vi "wayne.vi"() -> ()   [LabVIEW 2012]
uses:
  <vilib>/DAQmx/write.llb/DAQmx Write.vi
  <vilib>/DAQmx/write.llb/DAQmx Write (Digital 1D Bool NChan 1Samp 1Line).vi
  <vilib>/DAQmx/miscellaneous.llb/DAQmx Fill In Error Info.vi
  <vilib>/DAQmx/create/channels.llb/DAQmx Create Virtual Channel.vi
  <vilib>/DAQmx/create/channels.llb/DAQmx Create Channel (DO-Digital Output).vi
panel:
  out "inhibit":dbl=10.092000007629395
  out "delay":dbl=11.291999816894531
  in  "delay time (s)":dbl=1.2
  in  "Rolling Average Size":i32=25 min=1 step=1
  in  "inhibit time (s)":dbl=18.0
  in  "ECOLAB Button":bool
  in  "Tab Control":enum32{" GRAPHS   ", "CONFIG"}(tab)
  in  "on pulse simulator":bool
  out "Graph [0]":cluster{"Waveform":dbl, dbl}(graph)={"Waveform"=-0.0019147462699382683, -0.0017572258204325486}
  in  "on threshold (volts)":dbl=0.5
  out "AI":dbl[](array[numeric])=[-0.0017572258204325486] format="%.3f"
  out "DAQ Loop":i32=93368
  in  "DAQ wait ms":u32=3
  out "ON Pulse":bool
  in  "off threshold (volts)":dbl=-0.2
  in  "off pulse simulator":bool
  out "SOAP SIGNAL":bool
  out "Time (s)":dbl
  out "9205 Error":errorcluster
  in  "DAQ Selection":tag="9205/ai0"
  in  "maximum value":dbl=10.0
  in  "minimum value":dbl=-10.0
  out "9481 Error":errorcluster
  in  "9481 Name":tag="9481"
  in  "Relay Control":bool[](array[boolean])=[FALSE, FALSE, FALSE, FALSE]
  in  "Trim HI / LO [%]":dbl=2.0 min=0.0 max=100.0
  in  "Stop Program":bool=TRUE
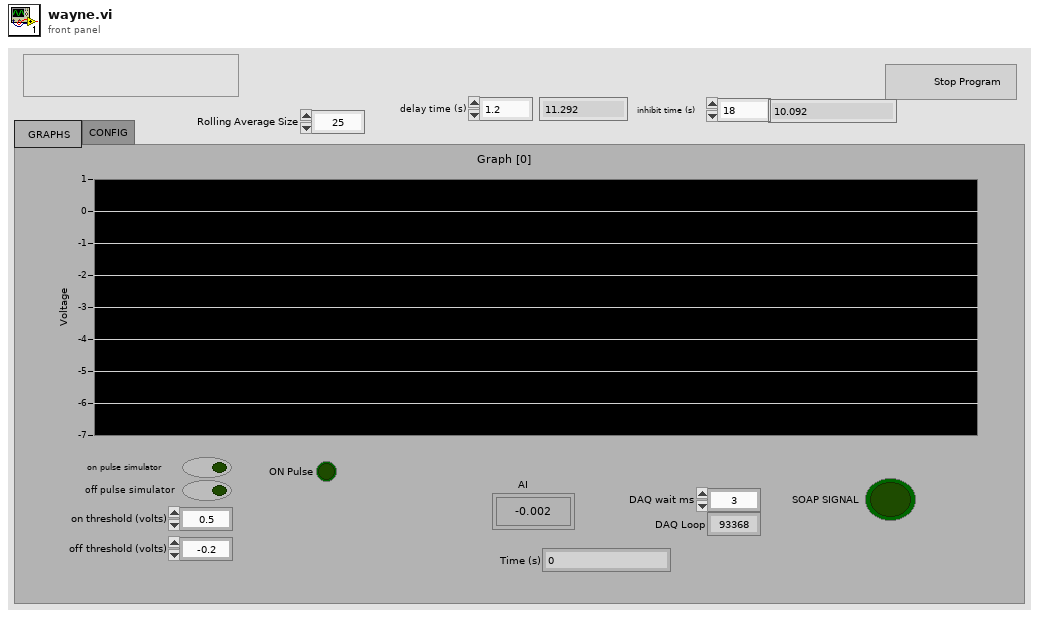
[diagram p1: front panel]
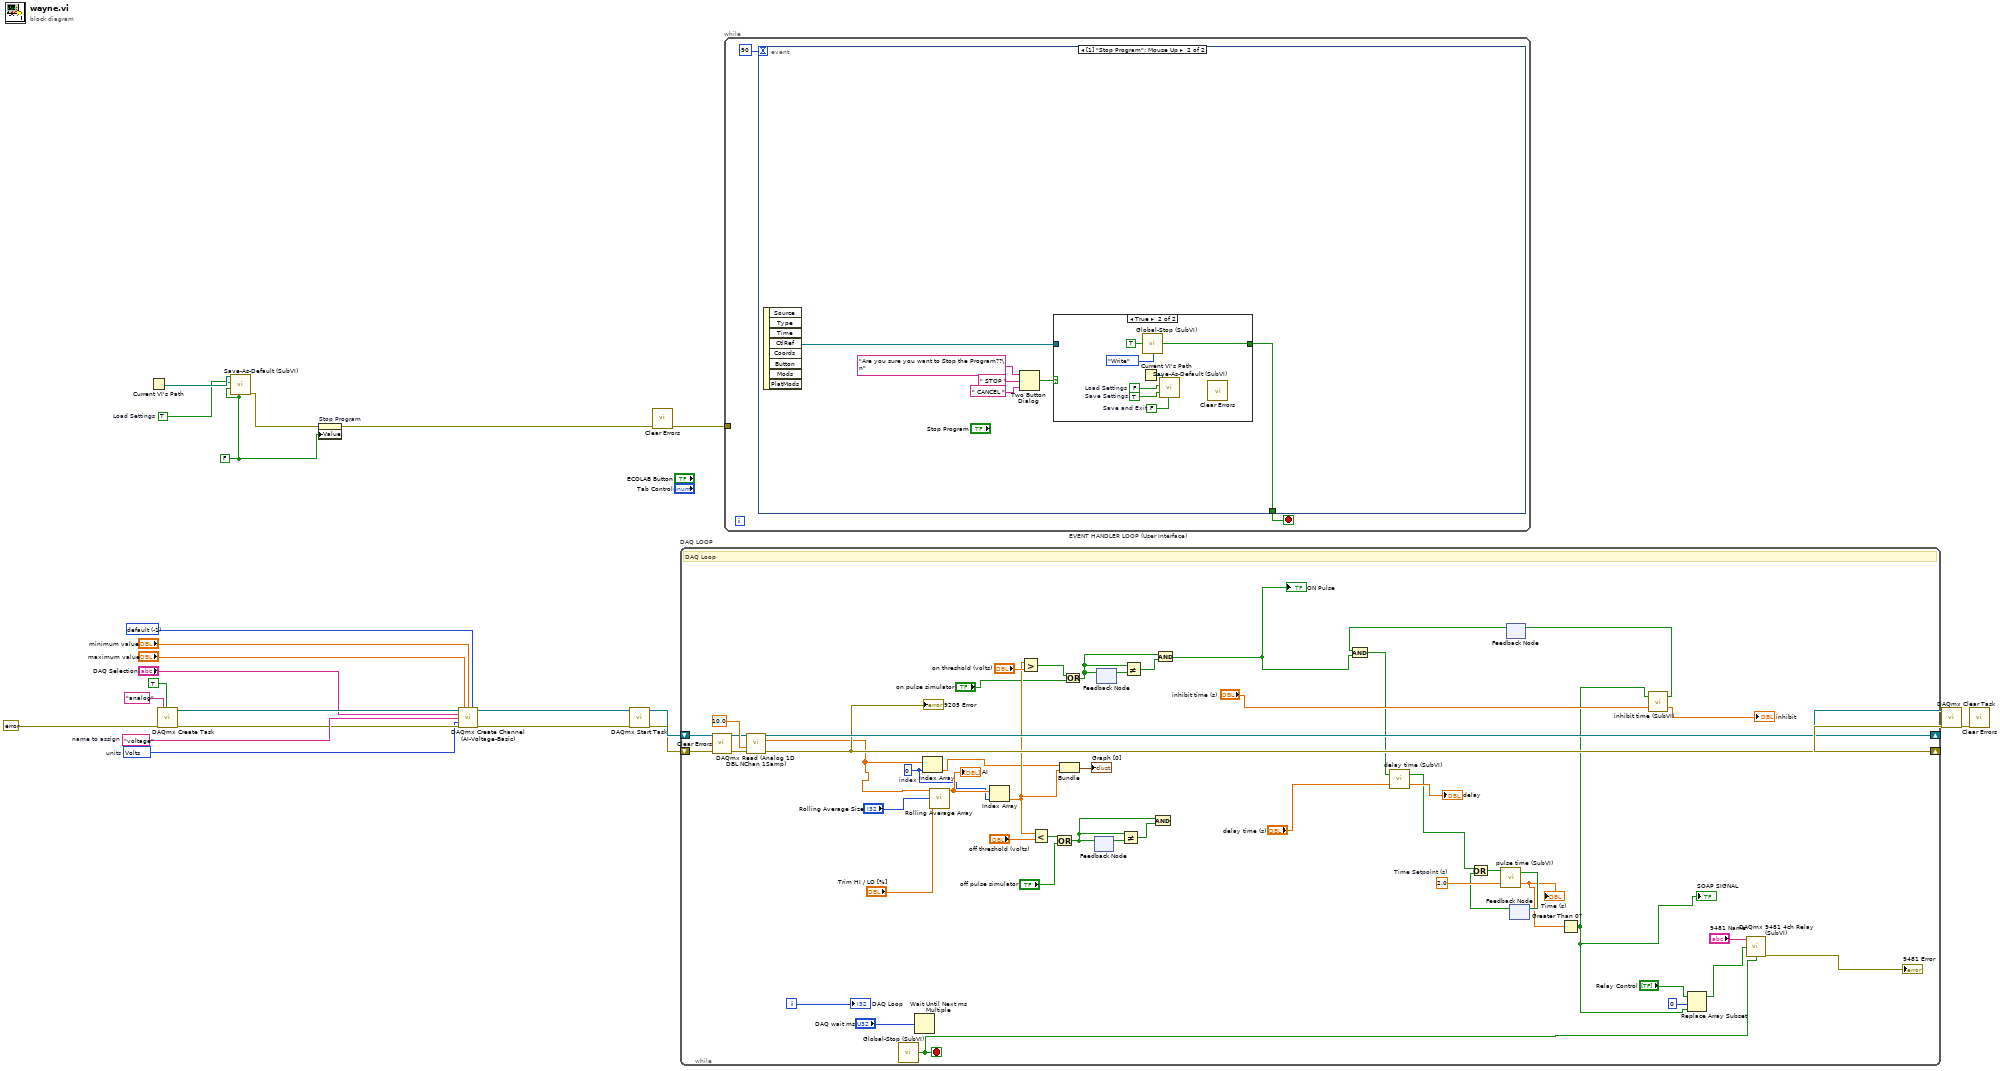
[diagram p0: block diagram]
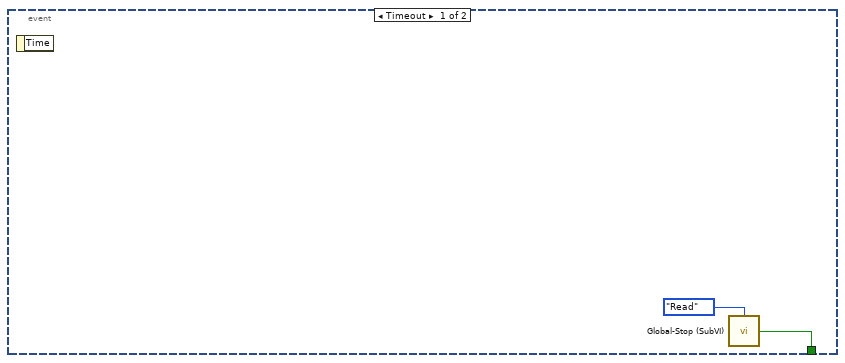
[diagram p2: hidden frame]
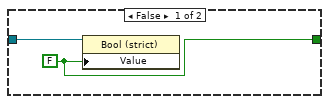
[diagram p3: hidden frame]
diagram:
  w3 = TRUE  # Load Settings
  w6 = 10348 items=["Volts"=10348, "From Custom Scale"=10065]  # units
  w8 = "voltage"  # name to assign
  w1 = FALSE
  w14 = -1 items=["default"=-1, "RSE"=10083, "NRSE"=10078, "Differential"=10106, "Pseudodifferential"=12529]
  n1 = Current VI's Path() -> (path=w4:path)
  n2 = call <vilib>:"DAQmx Create Task.vi"("new task name"="analog", "auto cleanup"=TRUE, "error in"=errorcluster {"status"=FALSE, "code"=0, "source"=""}) -> ("task out"=w13:refnum<k21>, "error out"=w7:errorcluster)  [unwired: 11 in]
  n3 = call "Save-As-Default (SubVI).vi"("Current VI's Path"=w4, "Load Settings"=w3, "Save Settings"=w1, "Save and Exit"=w1) -> ("Save as Default Error"=w2:errorcluster)  [unwired: 15 in]
  n4 = property on="Stop Program" class="Bool (strict)"(error in=w2, "Value"=w1) -> (error out=w17:errorcluster)  [unwired: 1 in, 1 out]
  n5 = call <vilib>:"DAQmx Create Channel (AI-Voltage-Basic).vi"("task in"=w13, "maximum value"="maximum value", "minimum value"="minimum value", "input terminal configuration"=w14, "physical channels"="DAQ Selection", "name to assign"=w8, "units"=w6, "error in"=w7) -> ("task out"=w10:refnum<k21>, "error out"=w9:errorcluster)  [unwired: 6 in]
  n6 = call <vilib>:"DAQmx Start Task.vi"("task/channels in"=w10, "error in"=w9) -> ("task out"=w20:refnum<k21>, "error out"=w18:errorcluster)  [unwired: 12 in]
  n7 = call <vilib>:"Clear Errors.vi"("error in (no error)"=w17) -> ("error out"=w16:errorcluster)  [unwired: 6 out]
  n8 = while "DAQ LOOP" {
    shift-right: [w68] -> w19
    shift-left: w20 -> [w70]
    shift-right: [w67] -> w22
    shift-left: w18 -> [w73]
    i -> [w58]
    stop <- w64 stop-if-true
    w35 = 2.0  # Time Setpoint (s)
    w47 = 0  # index
    # "DAQ Loop"
    n9 = call <vilib>:"Clear Errors.vi"("error in (no error)"=w73) -> ("error out"=w69:errorcluster)  [unwired: 6 in]
    n10 = call <vilib>:"DAQmx Read (Analog 1D DBL NChan 1Samp).vi"("task/channels in"=w70, "timeout"=10.0, "error in"=w69) -> ("task out"=w68:refnum<k21>, "data"=w48:dbl[], "error out"=w67:errorcluster)  [unwired: 10 in]
    "9205 Error" <- w67
    n11 = call "Global-Stop (SubVI).vi"() -> ("OUT"=w64:bool)  [unwired: 4 in]
    n12 = Wait Until Next ms Multiple(millisecond multiple="DAQ wait ms") -> ()  [unwired: 1 out]
    n13 = Index Array(array=w48, index=w47) -> (element=w44:dbl)
    n14 = call "Rolling Average Array.vi"("Raw Signals"=w48, "Rolling Average Size"="Rolling Average Size", "Trim HI / LO [%]"="Trim HI / LO [%]") -> ("Averaged Signals"=w49:dbl[])  [unwired: 12 in]
    "AI" <- w49
    n15 = Index Array(array=w49, index=w47) -> (element=w46:dbl)
    n16 = Greater?(x=w46, y="on threshold (volts)") -> (0:w41:bool)
    n17 = Less?(x=w46, y="off threshold (volts)") -> (x < y?=w54:bool)
    n18 = Or(x=w54, y="off pulse simulator") -> (x .or. y?=w52:bool)
    n19 = Bundle("Waveform"=w44, w46) -> (→"Graph [0]":cluster{"Waveform":dbl, dbl})  [unwired: 1 in]
    n20 = Or(x=w41, y="on pulse simulator") -> (x .or. y?=w40:bool)
    n21 = feedback #1() -> (w59:bool)  [unwired: 1 in]
    n22 = feedback-in #1(w52) -> ()
    n23 = feedback #2() -> (w62:bool)  [unwired: 1 in]
    n24 = feedback-in #2(w40) -> ()
    n25 = Not Equal?(x=w52, y=w59) -> (x != y?=w60:bool)
    n26 = Not Equal?(x=w40, y=w62) -> (x != y?=w43:bool)
    n27 = And(x=w52, y=w60) -> ()  [unwired: 1 out]
    n28 = And(x=w40, y=w43) -> (x .and. y?=w28:bool)
    "ON Pulse" <- w28
    n29 = feedback #3() -> (w26:bool)  [unwired: 1 in]
    n30 = And(x=w26, y=w28) -> (x .and. y?=w27:bool)
    n31 = call "delay time (SubVI).vi"("Time Setpoint (s)"="delay time (s)", "START/RESET TIMER"=w27) -> ("Time (s)"=→"delay":dbl, "Time Elapsed"=w33:bool)
    n32 = feedback #4() -> (w32:bool)  [unwired: 1 in]
    n33 = Or(x=w33, y=w32) -> (x .or. y?=w31:bool)
    n34 = call "pulse time (SubVI).vi"("Time Setpoint (s)"=w35, "START/RESET TIMER"=w31) -> ("Time (s)"=w30:dbl, "Time Elapsed"=w34:bool)
    "Time (s)" <- w30
    n35 = feedback-in #4(w34) -> ()
    n36 = Greater Than 0?(x=w30) -> (x > 0?=w25:bool)
    "SOAP SIGNAL" <- w25
    n37 = call "inhibit time (SubVI).vi"("Time Setpoint (s)"="inhibit time (s)", "START/RESET TIMER"=w25) -> ("Time (s)"=→"inhibit":dbl, "Time Elapsed"=w29:bool)
    n38 = feedback-in #3(w29) -> ()
    n39 = Replace Array Subset(array="Relay Control", new element=w25, index=0) -> (w55:bool[])
    n40 = call "DAQmx 9481 4ch Relay (SubVI).vi"("9481 Name"="9481 Name", "Relay Control"=w55, "Stop Program"=w64) -> ("9481 Error"=→"9481 Error":errorcluster)  [unwired: 12 in]
    "DAQ Loop" <- w58
  }
  n41 = while "EVENT HANDLER LOOP (User Interface)" {
    tunnel: w16 -> [_]
    stop <- w75 stop-if-true
    n42 = event shown="[1] \"Stop Program\": Mouse Up" {
      selector: _ -> [_ _]
      dyn-events: _ -> [_ _]
      timeout: 90 -> [_ _]
      tunnel: [w76 w79] -> w75
      event Timeout {
        n43 = event-data() -> ()  [unwired: 2 out]
        n44 = call "Global-Stop (SubVI).vi"("Mode (Read)"=enum16{"Read", "Write"}."Read") -> ("OUT"=w76:bool)  [unwired: 3 in]
      }
      event "Stop Program": Mouse Up {
        n45 = event-data() -> ("CtlRef"=w78:refnum<vi>)  [unwired: 8 out]
        n46 = Two Button Dialog(message="Are you sure you want to Stop the Program??\n", 1:" CANCEL " ("F button name (\"Cancel\")"), 2:" STOP ") -> (T button?=w80:bool)
        n47 = case shown="True" w80 {
          tunnel: [w84 w90] -> w79
          tunnel: w78 -> [w85 _]
          frame False {
            w84 = FALSE ("Value")
            n48 = property class="Bool (strict)"(reference=w85, "Value"=w84) -> ()  [unwired: 1 in, 2 out]
          }
          frame True {
            w86 = FALSE  # Save and Exit
            w87 = TRUE  # Save Settings
            w88 = FALSE  # Load Settings
            n49 = Current VI's Path() -> (path=w89:path)
            n50 = call "Global-Stop (SubVI).vi"("Mode (Read)"=enum16{"Read", "Write"}."Write", "IN"=TRUE) -> ("OUT"=w90:bool)  [unwired: 2 in]
            n51 = call "Save-As-Default (SubVI).vi"("Current VI's Path"=w89, "Load Settings"=w88, "Save Settings"=w87, "Save and Exit"=w86) -> ()  [unwired: 15 in, 1 out]
            n52 = call <vilib>:"Clear Errors.vi"() -> ()  [unwired: 1 in, 7 out]
          }
        }
      }
    }
  }
  n53 = call <vilib>:"DAQmx Clear Task.vi"("task in"=w19, "error in"=w22) -> ("error out"=w24:errorcluster)  [unwired: 13 out]
  n54 = call <vilib>:"Clear Errors.vi"("error in (no error)"=w24) -> ()  [unwired: 6 in, 1 out]
